vi "Create Steering Wheel.vi"(4 "steering motor communication":refnum<class "NI_Robotics_Motor Communication.lvclass">, 6 "motor communication":refnum<class "NI_Robotics_Motor Communication.lvclass">, 7 "steering parameters":T1={"steering gear ratio"=1.0, "motor angle offset (rad)"=0.0, "steering angle range"={"min steering angle (rad)"=-3.14159, "max steering angle (rad)"=3.141592653589793}}, 8 "error in (no error)":errorcluster, 10 "wheel name":string, 11 "wheel parameters":T3={"wheel radius"=1.0, "gear ratio"=1.0, "forward rotation direction"=0} {"forward rotation direction" items=["Clockwise", "Counterclockwise"]}) -> (0 "error out":errorcluster, 3 "steering wheel out":refnum<class "NI_Robotics_Steering Wheel.lvclass">)   [LabVIEW 2017, in "NI_Robotics_Steering Wheel.lvclass"]
doc: "Creates a wheel of the type you specify that you can add to a steering frame. You must manually select the polymorphic instance to use."
uses:
  <vilib>/robotics/Steering/Steering Wheel/NI_Robotics_Steering Wheel.lvclass
  c:/Program Files (x86)/National Instruments/LabVIEW 2017/vi.lib/robotics/Steering/Wheel/NI_Robotics_Wheel.lvclass
  <vilib>/robotics/Steering/Wheel/Wheel Parameters.ctl
  <vilib>/robotics/Steering/Wheel/Rotation Direction.ctl
  <vilib>/robotics/Actuation/Motor Communication/NI_Robotics_Motor Communication.lvclass
  <vilib>/robotics/Steering/Steering Wheel/Steering Wheel Parameters.ctl
  <vilib>/robotics/Steering/Steering Wheel/Steering Angle Range.ctl
  <vilib>/robotics/Actuation/Motor Communication/NI_Robotics_Motor Communication.lvclass/NI_Robotics_Motor Communication.ctl
  <vilib>/robotics/Steering/Wheel/NI_Robotics_Wheel.lvclass/NI_Robotics_Wheel.ctl
  <vilib>/robotics/Steering/Steering Wheel/NI_Robotics_Steering Wheel.lvclass/NI_Robotics_Steering Wheel.ctl
  <vilib>/robotics/Actuation/Motor Communication/Get Initialized State.vi
  <vilib>/robotics/Actuation/Motor Communication Val/NI_Robotics_Motor Communication Val.lvclass
  c:/Program Files (x86)/National Instruments/LabVIEW 2017/vi.lib/robotics/Actuation/Motor Communication/NI_Robotics_Motor Communication.lvclass
  <vilib>/robotics/Actuation/Motor Communication Val/Initialize Motor Communication Val.vi
  <vilib>/robotics/Steering/Wheel/NI_Robotics_Wheel.lvclass
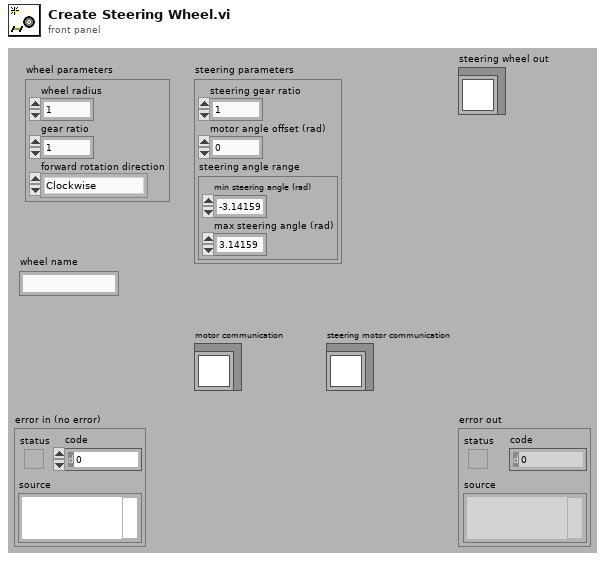
[diagram p1: front panel]
types:
  T1 = typedef "NI_Robotics_Steering Wheel.lvclass/Steering Wheel Parameters.ctl" = cluster{"steering gear ratio":dbl, "motor angle offset (rad)":dbl, "steering angle range":T2}
  T2 = typedef "NI_Robotics_Steering Wheel.lvclass/Steering Angle Range.ctl" = cluster{"min steering angle (rad)":dbl, "max steering angle (rad)":dbl}
  T3 = typedef "NI_Robotics_Wheel.lvclass/Wheel Parameters.ctl" = cluster{"wheel radius":dbl, "gear ratio":dbl, "forward rotation direction":T4}
  T4 = typedef "NI_Robotics_Wheel.lvclass/Rotation Direction.ctl" = u16
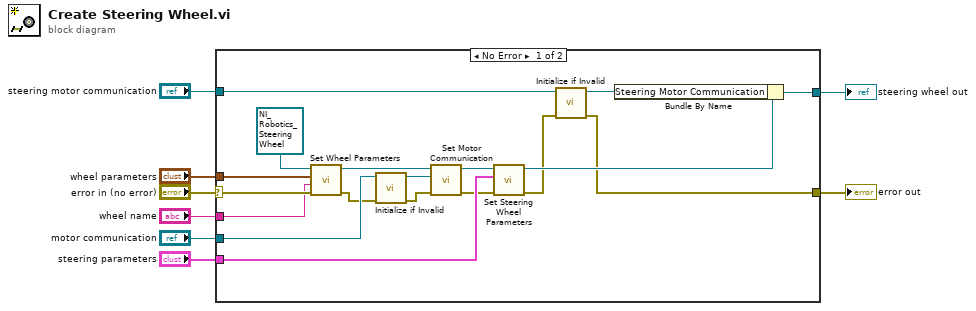
[diagram p0: block diagram]
diagram:
  n1 = case shown="No Error" "error in (no error)" {
    selector: "error in (no error)" -> [w24 w27]
    tunnel: [w9 w27] -> w7
    tunnel: "wheel parameters" -> [w25 _]
    tunnel: "motor communication" -> [w16 _]
    tunnel: "steering parameters" -> [w23 _]
    tunnel: "steering motor communication" -> [w12 _]
    tunnel: [w21 _] -> w2
    tunnel: "wheel name" -> [w20 _]
    frame No Error {
      n2 = call <vilib>:"Set Wheel Parameters.vi"("error in (no error)"=w24, "wheel name"=w20, "wheel parameters"=w25, "wheel in"=refnum<class "NI_Robotics_Steering Wheel.lvclass"> refnum ("SteeringWheel in")) -> ("error out"=w13:errorcluster, "wheel out"=w19:refnum<class "NI_Robotics_Steering Wheel.lvclass">)  [unwired: 6 in]
      n3 = call <vilib>:"Initialize if Invalid.vi"("error in (no error)"=w13, "motor communication in"=w16) -> ("error out"=w14:errorcluster, "motor communication out"=w15:refnum<class "NI_Robotics_Motor Communication.lvclass">)  [unwired: 7 in, 1 out]
      n4 = call <vilib>:"Set Motor Communication.vi"("error in (no error)"=w14, "motor communication"=w15, "wheel in"=w19) -> ("error out"=w17:errorcluster, "wheel out"=w18:refnum<class "NI_Robotics_Steering Wheel.lvclass">)  [unwired: 7 in]
      n5 = call <vilib>:"Set Steering Wheel Parameters.vi"("error in (no error)"=w17, "steering parameters"=w23, "steering wheel in"=w18) -> ("error out"=w10:errorcluster, "steering wheel out"=w22:refnum<class "NI_Robotics_Steering Wheel.lvclass">)  [unwired: 7 in]
      n6 = call <vilib>:"Initialize if Invalid.vi"("error in (no error)"=w10, "motor communication in"=w12) -> ("error out"=w9:errorcluster, "motor communication out"=w11:refnum<class "NI_Robotics_Motor Communication.lvclass">)  [unwired: 7 in, 1 out]
      n7 = Bundle By Name(cluster=w22, "Steering Motor Communication"=w11) -> (w21:refnum<class "NI_Robotics_Steering Wheel.lvclass">)
    }
    frame Error {
    }
  }
  "error out" <- w7
  "steering wheel out" <- w2
